vi "대한상공회의소 데이터셋 Test.vi"() -> ()   [LabVIEW 2020]
uses:
  <vilib>/DAQmx/read.llb/DAQmx Read (Analog 1D Wfm NChan NSamp).vi
  <vilib>/Analysis/baseanly.llb/Mean (DBL).vi
  <vilib>/DAQmx/create/channels.llb/DAQmx Create Channel (AI-Voltage-Basic).vi
  <vilib>/DAQmx/configure/timing.llb/DAQmx Timing (Sample Clock).vi
  <vilib>/DAQmx/miscellaneous.llb/DAQmx Fill In Error Info.vi
  <vilib>/Utility/file.llb/Write Delimited Spreadsheet (DBL).vi
  <vilib>/Analysis/NI_AALBase.lvlib
panel:
  out "x = y?":bool
  out "Python Class":string
  out "숫자":i32
  in  "IR 하위 리미트":dbl=1.0 format="%#_13g"
  in  "IR 상위 리미트":dbl=2.8 format="%#_13g"
  in  "기울기Y 하위 리미트":dbl=-8.0 format="%#_13g"
  in  "기울기Y 상위 리미트":dbl=-2.0 format="%#_13g"
  in  "기울기X 하위 리미트":dbl=-10.0 format="%#_13g"
  in  "기울기X 상위 리미트":dbl=-4.0 format="%#_13g"
  in  "가속도 하위 리미트":dbl=0.09 format="%#_13g"
  in  "가속도 상위 리미트":dbl=0.27 format="%#_13g"
  out "Class":string
  out "출력 클러스터":cluster{dbl, dbl, dbl, dbl}(graph)
  in  "정지":bool
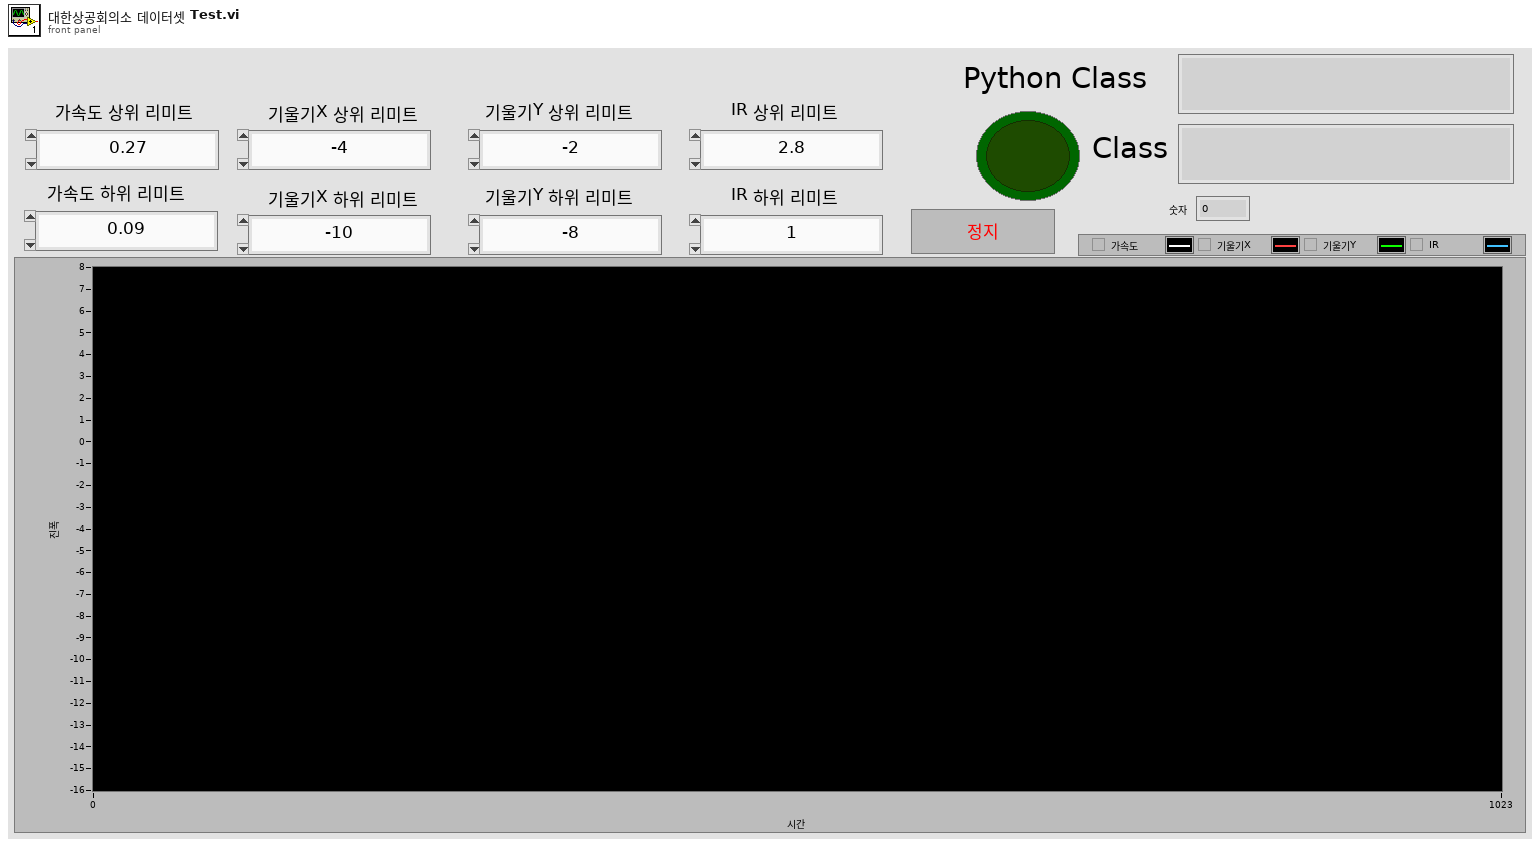
[diagram p1: front panel]
types:
  T1 = enum16{"Standard", "Buffered", "CRLF", "Immediate"}
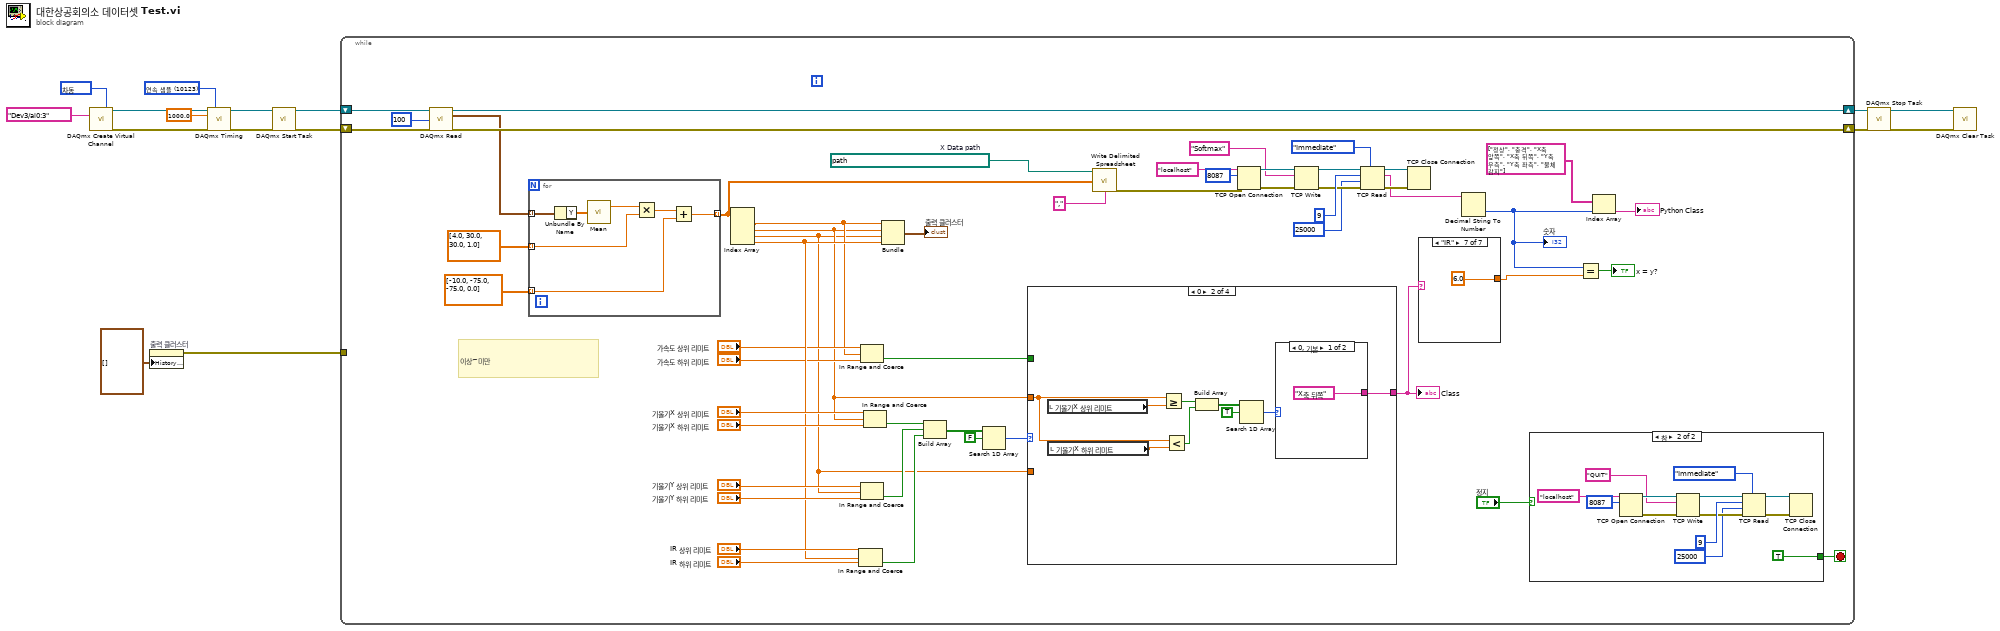
[diagram p0: block diagram]
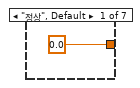
[diagram p3: hidden frame]
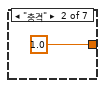
[diagram p4: hidden frame]
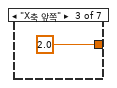
[diagram p5: hidden frame]
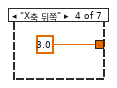
[diagram p6: hidden frame]
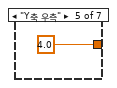
[diagram p7: hidden frame]
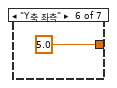
[diagram p8: hidden frame]
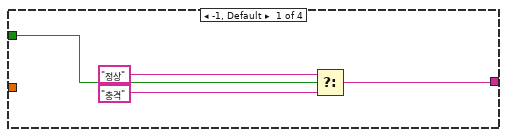
[diagram p9: hidden frame]
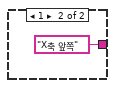
[diagram p10: hidden frame]
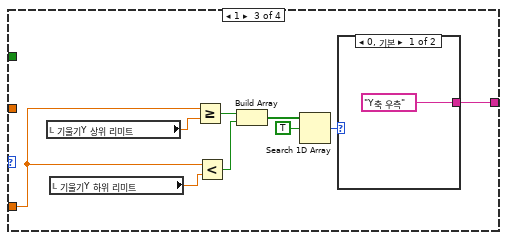
[diagram p11: hidden frame]
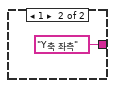
[diagram p12: hidden frame]
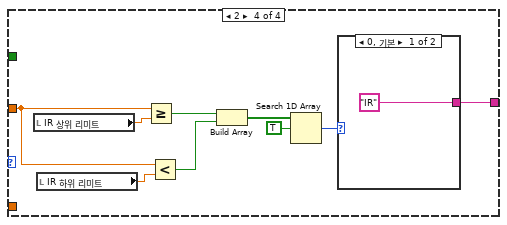
[diagram p13: hidden frame]
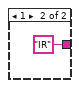
[diagram p14: hidden frame]
diagram:
  w4 = 10123 items=["유한 샘플"=10178, "연속 샘플"=10123, "하드웨어 타이밍에 의한 단일 포인트"=12522] ("sample mode")
  w5 = 10106 items=["기본"=-1, "RSE"=10083, "NRSE"=10078, "차동"=10106, "유사 차동"=12529] ("input terminal configuration")
  n1 = call-poly <vilib>:"DAQmx Create Virtual Channel.vi"("input terminal configuration"=w5, "physical channels"=tag "Dev3/ai0:3") -> ("task out"=w16:refnum<k21>, "error out"=w15:errorcluster)  [unwired: 12 in]
  n2 = property on="출력 클러스터" class="WFChart (엄격한)"("History Data"=cluster{dbl, dbl, dbl, dbl}[] [] ("히스토리 데이터")) -> (error out=w1:errorcluster)  [unwired: 2 in, 1 out]
  n3 = call-poly <vilib>:"DAQmx Timing.vi"("task/channels in"=w16, "sample mode"=w4, "rate"=1000.0, "error in"=w15) -> ("task out"=w14:refnum<k21>, "error out"=w13:errorcluster)  [unwired: 10 in]
  n4 = call <vilib>:"DAQmx Start Task.vi"("task/channels in"=w14, "error in"=w13) -> ("task out"=w12:refnum<k21>, "error out"=w11:errorcluster)  [unwired: 12 in]
  n5 = while {
    shift-right: [w67] -> w10
    shift-left: w12 -> [w69]
    shift-right: [w66] -> w9
    shift-left: w11 -> [w68]
    tunnel: w1 -> [_]
    stop <- w23 stop-if-true
    w41 = path "C:/Users/유현재/Desktop/est4.csv"  # X Data path
    # "이상~미만"
    n6 = call-poly <vilib>:"DAQmx Read.vi"("task/channels in"=w69, "number of samples per channel"=100, "error in"=w68) -> ("task out"=w67:refnum<k21>, "data"=w61:waveform(dbl)[], "error out"=w66:errorcluster)  [unwired: 10 in]
    n7 = for {
      tunnel: w61 -> [w133] mode=indexing
      tunnel: dbl[] [4.0, 30.0, 30.0, 1.0] -> [w128] mode=indexing
      tunnel: dbl[] [-10.0, -75.0, -75.0, 0.0] -> [w127] mode=indexing
      tunnel: [w130] -> w38 mode=indexing
      n8 = Unbundle By Name(w133) -> ("Y"=w129:dbl[])
      n9 = call-poly <vilib>:"Mean.vi"("X"=w129) -> ("mean"=w131:dbl)  [unwired: 1 out]
      n10 = Multiply(x=w131, y=w128) -> (x*y=w132:dbl)
      n11 = Add(x=w132, y=w127) -> (x+y=w130:dbl)
    }
    n12 = Index Array(array=w38) -> (element #1=w45:dbl, element #2=w43:dbl, element #3=w42:dbl, element #4=w54:dbl)  [unwired: 4 in]
    n13 = In Range and Coerce(upper limit="IR 상위 리미트", x=w54, lower limit="IR 하위 리미트") -> (In Range?=w51:bool)  [unwired: 1 out]
    n14 = In Range and Coerce(upper limit="가속도 상위 리미트", x=w45, lower limit="가속도 하위 리미트") -> (In Range?=w44:bool)  [unwired: 1 out]
    n15 = In Range and Coerce(upper limit="기울기Y 상위 리미트", x=w42, lower limit="기울기Y 하위 리미트") -> (In Range?=w52:bool)  [unwired: 1 out]
    n16 = In Range and Coerce(upper limit="기울기X 상위 리미트", x=w43, lower limit="기울기X 하위 리미트") -> (In Range?=w53:bool)  [unwired: 1 out]
    n17 = Bundle(w45, w43, w42, w54) -> (→"출력 클러스터":cluster{dbl, dbl, dbl, dbl})  [unwired: 1 in]
    n18 = Build Array(w53, w52, w51) -> (w50:bool[])
    n19 = Search 1D Array(1D array=w50, element=FALSE ("원소")) -> (index of element=w48:i32)  [unwired: 1 in]
    n20 = case shown="0" w48 {
      tunnel: w44 -> [w93 _ _ _]
      tunnel: [w90 w97 w108 w118] -> w40
      tunnel: w43 -> [_ w96 _ w124]
      tunnel: w42 -> [_ _ w107 _]
      frame -1, Default {
        n21 = Select(t="정상", s=w93, f="충격") -> (s? t:f=w90:string)
      }
      frame 0 {
        n22 = local read "기울기X 상위 리미트"() -> (w94:dbl)
        n23 = local read "기울기X 하위 리미트"() -> (w95:dbl)
        n24 = Greater Or Equal?(x=w96, y=w94) -> (x >= y?=w102:bool)
        n25 = Less?(x=w96, y=w95) -> (x < y?=w101:bool)
        n26 = Build Array(w102, w101) -> (w100:bool[])
        n27 = Search 1D Array(1D array=w100, element=TRUE ("원소")) -> (index of element=w98:i32)  [unwired: 1 in]
        n28 = case shown="0, 기본" w98 {
          tunnel: ["X축 뒤쪽" "X축 앞쪽"] -> w97
          frame 0, Default {
          }
          frame 1 {
          }
        }
      }
      frame 1 {
        n29 = local read "기울기Y 상위 리미트"() -> (w106:dbl)
        n30 = local read "기울기Y 하위 리미트"() -> (w105:dbl)
        n31 = Greater Or Equal?(x=w107, y=w106) -> (x >= y?=w113:bool)
        n32 = Less?(x=w107, y=w105) -> (x < y?=w112:bool)
        n33 = Build Array(w113, w112) -> (w111:bool[])
        n34 = Search 1D Array(1D array=w111, element=TRUE ("원소")) -> (index of element=w109:i32)  [unwired: 1 in]
        n35 = case shown="0, 기본" w109 {
          tunnel: ["Y축 우측" "Y축 좌측"] -> w108
          frame 0, Default {
          }
          frame 1 {
          }
        }
      }
      frame 2 {
        n36 = local read "IR 상위 리미트"() -> (w117:dbl)
        n37 = local read "IR 하위 리미트"() -> (w116:dbl)
        n38 = Greater Or Equal?(x=w124, y=w117) -> (x >= y?=w123:bool)
        n39 = Less?(x=w124, y=w116) -> (x < y?=w122:bool)
        n40 = Build Array(w123, w122) -> (w121:bool[])
        n41 = Search 1D Array(1D array=w121, element=TRUE ("원소")) -> (index of element=w119:i32)  [unwired: 1 in]
        n42 = case shown="0, 기본" w119 {
          tunnel: ["IR" "IR"] -> w118
          frame 0, Default {
          }
          frame 1 {
          }
        }
      }
    }
    "Class" <- w40
    n43 = call-poly <vilib>:"Write Delimited Spreadsheet.vi"("file path (dialog if empty)"=w41, "1D data"=w38, "delimiter (\\t)"="," ("delimiter (\\t)")) -> ("error out"=w27:errorcluster)  [unwired: 11 in, 1 out]
    n44 = TCP Open Connection(address="localhost", remote port or service name=u16 8087 ("원격 포트 또는 서비스 이름"), error in (no error)=w27) -> (connection ID=w32:refnum<k5>, error out=w31:errorcluster)  [unwired: 2 in]
    n45 = TCP Write(connection ID=w32, data in="Softmax" ("데이터 입력"), error in (no error)=w31) -> (connection ID out=w36:refnum<k5>, error out=w35:errorcluster)  [unwired: 1 in, 1 out]
    n46 = TCP Read(connection ID=w36, bytes to read=9, error in (no error)=w35, 7:T1."Immediate" ("모드(standard)"), 9:25000 ("timeout ms (25000)")) -> (connection ID out=w30:refnum<k5>, data out=w22:string, error out=w29:errorcluster)
    n47 = TCP Close Connection(connection ID=w30, error in (no error)=w29) -> ()  [unwired: 1 in, 2 out]
    n48 = case shown="\"IR\"" w40 {
      tunnel: [0.0 1.0 2.0 3.0 4.0 5.0 6.0] -> w19
      frame "정상", Default {
      }
      frame "충격" {
      }
      frame "X축 앞쪽" {
      }
      frame "X축 뒤쪽" {
      }
      frame "Y축 우측" {
      }
      frame "Y축 좌측" {
      }
      frame "IR" {
      }
    }
    n49 = Decimal String To Number(string=w22) -> (number=w18:i32)  [unwired: 2 in, 1 out]
    "숫자" <- w18
    n50 = case shown="참" "정지" {
      tunnel: [_ TRUE] -> w23
      frame False {
      }
      frame True {
        n51 = TCP Open Connection(address="localhost", remote port or service name=u16 8087 ("원격 포트 또는 서비스 이름")) -> (connection ID=w77:refnum<k5>, error out=w76:errorcluster)  [unwired: 3 in]
        n52 = TCP Write(connection ID=w77, data in="QUIT" ("데이터 입력"), error in (no error)=w76) -> (connection ID out=w81:refnum<k5>, error out=w80:errorcluster)  [unwired: 1 in, 1 out]
        n53 = TCP Read(connection ID=w81, bytes to read=9, error in (no error)=w80, 7:T1."Immediate" ("모드(standard)"), 9:25000 ("timeout ms (25000)")) -> (connection ID out=w75:refnum<k5>, error out=w74:errorcluster)  [unwired: 1 out]
        n54 = TCP Close Connection(connection ID=w75, error in (no error)=w74) -> ()  [unwired: 1 in, 2 out]
      }
    }
    n55 = Equal?(x=w18, y=w19) -> (x = y?=→"x = y?":bool)
    n56 = Index Array(array=string[] ["정상", "충격", "X축 앞쪽", "X축 뒤쪽", "Y축 우측", "Y축 좌측", "물체 감지"], index=w18) -> (element=→"Python Class":string)
  }
  n57 = call <vilib>:"DAQmx Stop Task.vi"("task/channels in"=w10, "error in"=w9) -> ("task out"=w8:refnum<k21>, "error out"=w7:errorcluster)  [unwired: 12 in]
  n58 = call <vilib>:"DAQmx Clear Task.vi"("task in"=w8, "error in"=w7) -> ()  [unwired: 13 in, 1 out]
